vi "FLip BMP.vi"(11 "data":u8[](array[numeric])=array[240054 elements]) -> (1 "Blank Image":bool, 3 "Array":u8[](array[numeric]))   [LabVIEW 2017]
panel:
  out "x*y":i32
  out "size(s)":i32
  out "output array":u8[][](array[numeric])
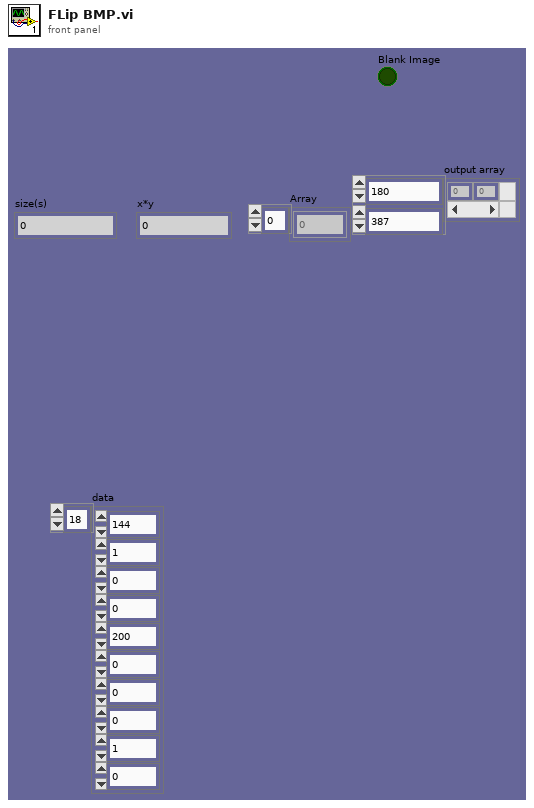
[diagram p1: front panel]
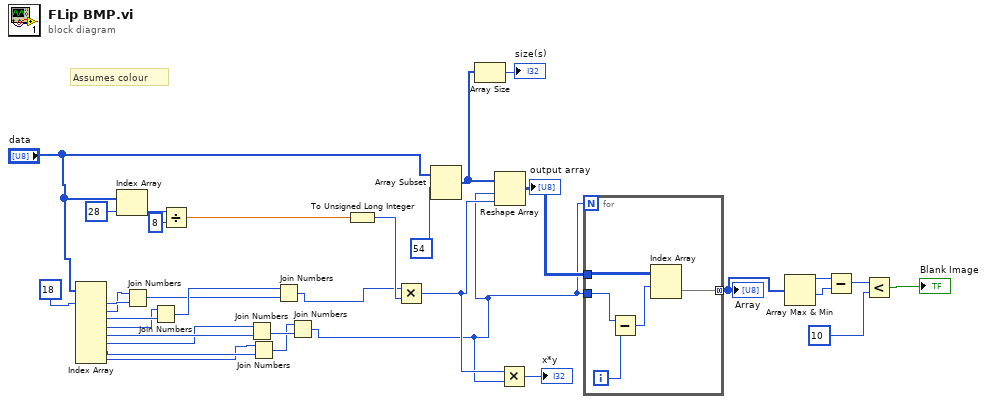
[diagram p0: block diagram]
diagram:
  # "Assumes colour"
  n1 = Index Array(array="data", index #1=18 ("index")) -> (element #1=w20:u8, element #2=w19:u8, element #3=w18:u8, element #4=w17:u8, element #5=w11:u8, element #6=w10:u8, element #7=w9:u8, element #8=w8:u8)  [unwired: 7 in]
  n2 = Index Array(array="data", index=28) -> (element=w26:u8)
  n3 = Join Numbers(hi=w19, lo=w20) -> ((hi.lo)=w15:u16)
  n4 = Join Numbers(hi=w17, lo=w18) -> ((hi.lo)=w16:u16)
  n5 = Divide(x=w26, y=u8 8) -> (x/y=w24:dbl)
  n6 = Join Numbers(hi=w10, lo=w11) -> ((hi.lo)=w13:u16)
  n7 = Join Numbers(hi=w8, lo=w9) -> ((hi.lo)=w12:u16)
  n8 = Join Numbers(hi=w16, lo=w15) -> ((hi.lo)=w14:u32)
  n9 = Join Numbers(hi=w12, lo=w13) -> ((hi.lo)=w7:u32)
  n10 = To Unsigned Long Integer(number=w24) -> (unsigned 32bit integer=w23:u32)
  n11 = Multiply(x=w14, y=w23) -> (x*y=w28:u32)
  n12 = Array Subset(array="data", index=54) -> (w31:u8[])  [unwired: 1 in]
  n13 = Array Size(array=w31) -> (size(s)=→"size(s)":i32)
  n14 = Reshape Array(w31, w7, w28) -> (w32:u8[][])
  "output array" <- w32
  n15 = Multiply(x=w28, y=w7) -> (x*y=→"x*y":u32)
  n16 = for {
    N: w7 -> [_]
    tunnel: w32 -> [w38]
    tunnel: [w35] -> w6 mode=concatenating
    tunnel: w7 -> [w34]
    i -> [w37]
    n17 = Subtract(x=w34, y=w37) -> (x-y=w36:u32)
    n18 = Index Array(array=w38, index (row)=w36) -> (element=w35:u8[])  [unwired: 1 in]
  }
  "Array" <- w6
  n19 = Array Max & Min(array=w6) -> (max value=w5:u8, min value=w4:u8)  [unwired: 2 out]
  n20 = Subtract(x=w5, y=w4) -> (x-y=w3:u8)
  n21 = Less?(x=w3, y=u8 10) -> (x < y?=→"Blank Image":bool)
